vi "CLR.vi"(0 "System no.":i32=1 min=1 max=4 step=1, 2 "CLR axes":string[](array[string]), 3 "All axes?":bool, 4 "Axis identifier?":bool=TRUE, 5 "error in":errorcluster) -> (19 "error out":errorcluster)   [LabVIEW 2020]
doc: "Clears axis status for specified axes.\n\nC-702: If All axes = TRUE, then Axis identifier must be TRUE\nC-843: If All axes = TRUE, then Axis identifier must be TRUE\nC-843.PM: If All axes = TRUE, then Axis identifier must be TRUE\nC-848: If All axes = TRUE, then Axis identifier must be TRUE\nC-865: If All axes = TRUE, then Axis identifier must be TRUE\nC-866: If All axes = TRUE, then Axis identifier must be TRUE\nC-880: If All axes = TRUE, then Axis identifier must be TRUE\nE-755: If All axes? = TRUE, then Axis identifier? must be TRUE"
panel:
  # "Clear axis status for specified axes."
  # "If all axes: use"
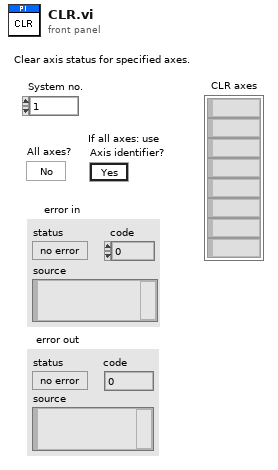
[diagram p1: front panel]
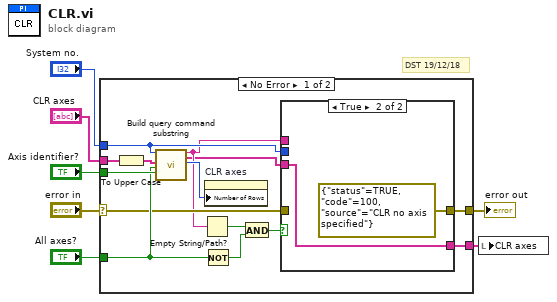
[diagram p0: block diagram]
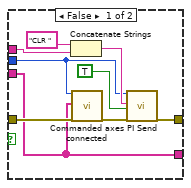
[diagram p2: hidden frame]
diagram:
  # "DST 19/12/18"
  n1 = case shown="No Error" "error in" {
    selector: "error in" -> [w13 w33]
    tunnel: "CLR axes" -> [w21 w34]
    tunnel: "Axis identifier?" -> [w19 _]
    tunnel: "System no." -> [w18 _]
    tunnel: "All axes?" -> [w16 _]
    tunnel: [w14 w33] -> w3
    tunnel: [w8 w34] -> w2
    frame No Error {
      n2 = To Upper Case(1:w21) -> (0:w20:string[])
      n3 = call "Build query command substring.vi"("System no."=w18, "Axes to query in"=w20, "Query\nAll axes?"=w16, "For all axes: use\nAxis identifier?"=w19) -> ("Command substring"=w12:string, "Axes to query out"=w9:string[], "Number of rows"=w17:u32)  [unwired: 2 in, 11 out]
      n4 = Empty String/Path?(string/path=w12) -> (empty?=w11:bool)
      n5 = Not(x=w16) -> (.not. x?=w15:bool)
      n6 = property on="CLR axes" class="Arr (strict)"("Number of Rows"=w17) -> ()  [unwired: 2 in, 2 out]
      n7 = And(x=w11, y=w15) -> (x .and. y?=w10:bool)
      n8 = case shown="True" w10 {
        tunnel: w18 -> [w27 _]
        tunnel: [w25 errorcluster {"status"=TRUE, "code"=100, "source"="CLR no axis specified"} ("error out")] -> w14
        tunnel: w9 -> [w22 w31]
        tunnel: w13 -> [w24 _]
        tunnel: w12 -> [w23 _]
        tunnel: [w22 w31] -> w8
        frame False {
          n9 = Concatenate Strings("CLR ", w23) -> (w28:string)
          n10 = call "Commanded axes connected.vi"("System no."=w27, "Commanded axes"=w22, "error in"=w24) -> ("error out"=w26:errorcluster)  [unwired: 1 in, 15 out]
          n11 = call "PI Send.vi"("System no."=w27, "String to send"=w28, "Attach termination char.?"=TRUE ("Attach Linefeed?"), "error in"=w26) -> ("error out"=w25:errorcluster)  [unwired: 2 in, 13 out]
        }
        frame True {
        }
      }
    }
    frame Error {
    }
  }
  "error out" <- w3
  n12 = local write "CLR axes"(w2) -> ()
